vi "Save Image.vi"(8 "Data":dbl[][](array[numeric]), 10 "Process Index":u8, 11 "Current File Num":u16) -> ()   [LabVIEW 2013]
panel:
  out "Path":path
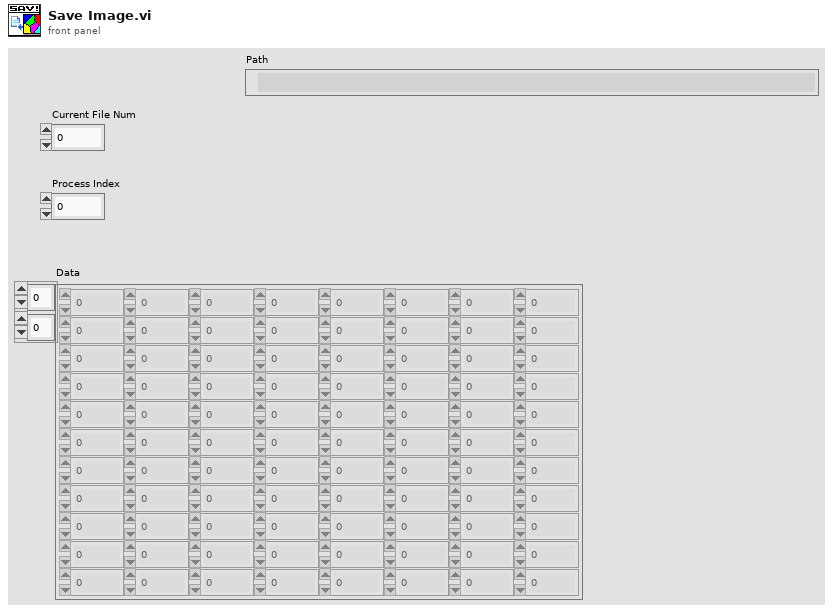
[diagram p1: front panel]
types:
  T1 = typedef "Image Type" = u32
  T2 = typedef "IMAQ Image.ctl" = refnum<image>
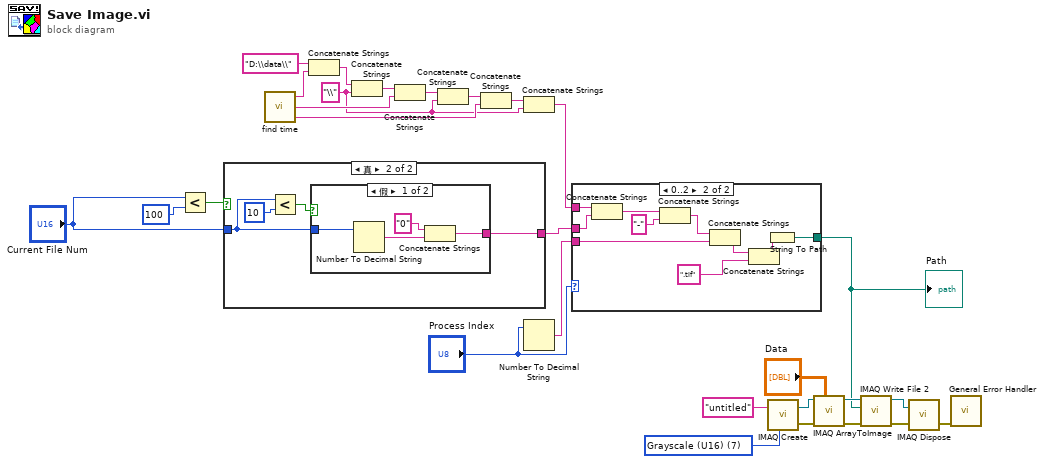
[diagram p0: block diagram]
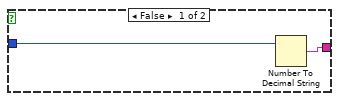
[diagram p2: hidden frame]
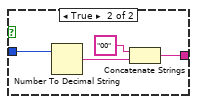
[diagram p3: hidden frame]
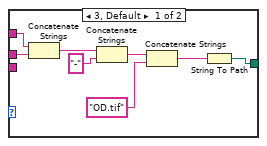
[diagram p4: hidden frame]
diagram:
  w9 = "\\" ("字符串")
  w21 = T1 7 items=["Grayscale (U8)", "Grayscale (I16)", "Grayscale (SGL)", "Complex (CSG)", "RGB (U32)", "HSL (U32)", "RGB (U64)", "Grayscale (U16)"] ("Image Type")
  n1 = Less?(x="Current File Num", y=u16 100) -> (x < y?=w1:bool)
  n2 = case shown="真" w1 {
    tunnel: "Current File Num" -> [w30 w32]
    tunnel: [w29 w31] -> w7
    frame False {
      n3 = Number To Decimal String(number=w30) -> (decimal integer string=w29:string)  [unwired: 1 in]
    }
    frame True {
      n4 = Less?(x=w32, y=u16 10) -> (x < y?=w33:bool)
      n5 = case shown="假" w33 {
        tunnel: w32 -> [w37 w42]
        tunnel: [w35 w39] -> w31
        frame False {
          n6 = Number To Decimal String(number=w37) -> (decimal integer string=w36:string)  [unwired: 1 in]
          n7 = Concatenate Strings("0" ("字符串"), w36) -> (w35:string)
        }
        frame True {
          n8 = Number To Decimal String(number=w42) -> (decimal integer string=w40:string)  [unwired: 1 in]
          n9 = Concatenate Strings("00" ("字符串"), w40) -> (w39:string)
        }
      }
    }
  }
  n10 = call "find time.vi"() -> ("day"=w11:string, "month"=w14:string, "year"=w17:string)  [unwired: 3 in]
  n11 = Concatenate Strings("D:\\data\\", w17) -> (w16:string)
  n12 = Concatenate Strings(w16, w9) -> (w15:string)
  n13 = Concatenate Strings(w15, w14) -> (w13:string)
  n14 = Concatenate Strings(w13, w9) -> (w12:string)
  n15 = Concatenate Strings(w12, w11) -> (w10:string)
  n16 = Concatenate Strings(w10, w9) -> (w6:string)
  n17 = Number To Decimal String(number="Process Index") -> (decimal integer string=w8:string)  [unwired: 1 in]
  n18 = case shown="0..2" "Process Index" {
    tunnel: [w44 w60] -> w5
    tunnel: w7 -> [w47 w59]
    tunnel: w8 -> [_ w55]
    tunnel: w6 -> [w43 w54]
    frame 3, Default {
      n19 = Concatenate Strings(w43, w47) -> (w50:string)
      n20 = Concatenate Strings(w50, "-" ("字符串")) -> (w48:string)
      n21 = Concatenate Strings(w48, "OD.tif" ("字符串")) -> (w45:string)
      n22 = String To Path(string=w45) -> (path=w44:path)
    }
    frame 0..2 {
      n23 = Concatenate Strings(w54, w59) -> (w58:string)
      n24 = Concatenate Strings(w58, "-" ("字符串")) -> (w56:string)
      n25 = Concatenate Strings(w56, w55) -> (w53:string)
      n26 = Concatenate Strings(w53, ".tif" ("字符串")) -> (w51:string)
      n27 = String To Path(string=w51) -> (path=w60:path)
    }
  }
  "Path" <- w5
  n28 = call "IMAQ Create"("Image Name"="untitled", "Image Type"=w21) -> ("New Image"=w19:T2, "error out"=w20:errorcluster)  [unwired: 3 in]
  n29 = call "IMAQ ArrayToImage"("Image Pixels (U16)"="Data", "error in (no error)"=w20, "Image"=w19) -> ("error out"=w24:errorcluster, "Image Out"=w27:T2)  [unwired: 7 in]
  n30 = call-poly "IMAQ Write File 2"("error in (no error)"=w24, "File Path"=w5, "Image"=w27) -> ("error out"=w25:errorcluster, "Image Out (duplicate)"=w26:T2)  [unwired: 7 in]
  n31 = call "IMAQ Dispose"("Image"=w26, "error in (no error)"=w25) -> ("error out"=w22:errorcluster)  [unwired: 4 in]
  n32 = call <vilib>:"General Error Handler.vi"("error in (no error)"=w22) -> ()  [unwired: 10 in, 5 out]
